vi "HostExample.vi"() -> ()   [LabVIEW 2023]
uses:
  <vilib>/FPGAPlugInAG/Dynamic/niLvFpga_Download_Dynamic.vi
  <vilib>/FPGAPlugInAG/Dynamic/niLvFpga_Run_Dynamic.vi
  <vilib>/LabVIEW Targets/FPGA/RIO/NiFpga_HostInterfaceExtensions/HdlFifo/NiFpga_HdlFifo_AddI32.vi
  API/HdlFifo/private/_NiFpga_HdlFifo_GetStream.vi
  <vilib>/Utility/error.llb/Error Cluster From Error Code.vi
  <vilib>/rvi/interface/nirviMethod/nirviMethod.xnode
  <vilib>/LabVIEW Targets/FPGA/RIO/NiFpga_HostInterfaceExtensions/HdlFifo/NiFpga_HdlFifo_WriteI32.vi
  <vilib>/LabVIEW Targets/FPGA/RIO/NiFpga_HostInterfaceExtensions/HdlFifo/NiFpga_HdlFifo_ReadI32.vi
panel:
  out "empty elements remaining":u64
  out "Elements Remaining":u64
  out "error out 6":errorcluster
  in  "WriteScratch":bool
  in  "ReadScratch":bool
  out "Scratch Read":u32 format="%.0x"
  in  "Scratch Write":u32 format="%.0x"
  in  "Num Elements":i32
  out "Read Data":u32[](array[numeric])
  in  "Read FPGA FIFO":bool
  in  "Write FPGA FIFO":bool
  in  "Write Data":u32[](array[numeric])
  in  "WriteReg":bool
  in  "ReadReg":bool
  out "Read Value":u32
  in  "Write Value":u32 format="%.0x"
  in  "Write Offset":u32
  in  "Read Offset":u32
  in  "Num Elements":i32
  out "Data 4":i32[](array[numeric])
  in  "Write Data":i32[](array[numeric])
  in  "Read Host FIFO":bool
  in  "Write Host FIFO":bool
  out "Numeric":i32
  in  "stop":bool
  # "Write and read any register offset"
  # "Write and read the scratch register"
  # "Scratch Register"
  # "Write and read the Host to FPGA FIFO"
  # "Host to FPGA FIFO"
  # "Write and read the FPGA to Host FIFO"
  # "FPGA to Host FIFO"
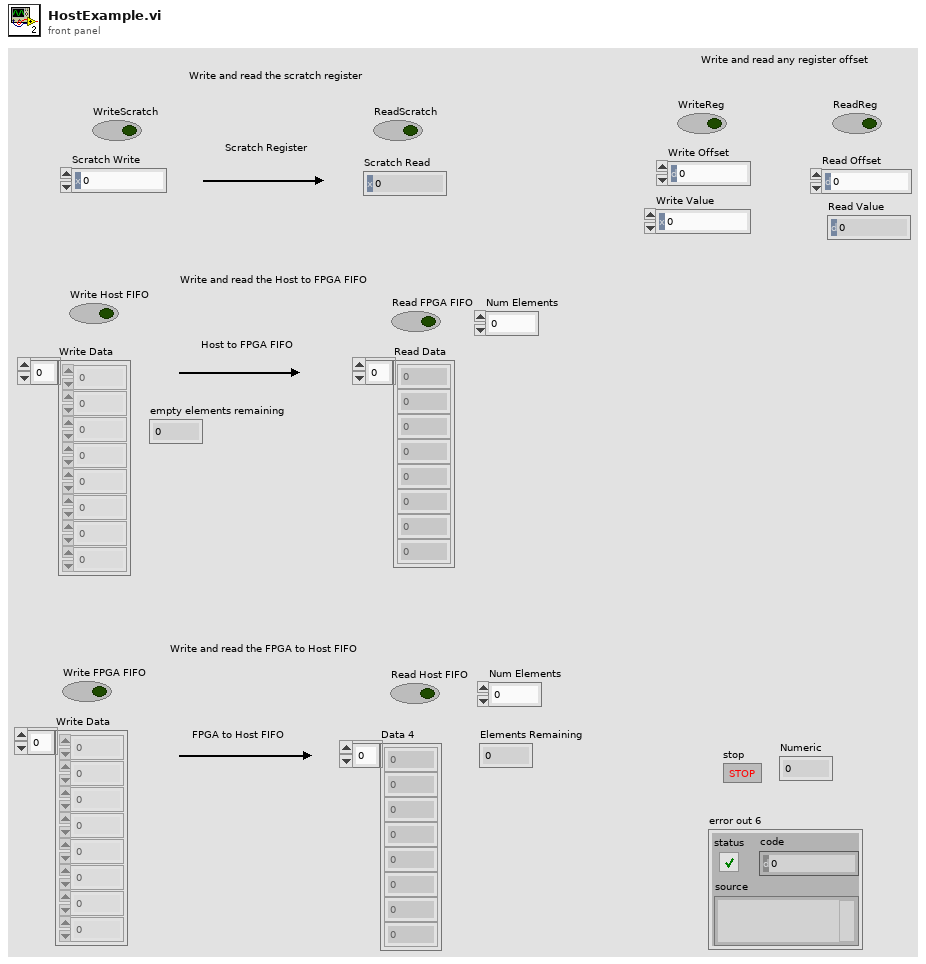
[diagram p1: front panel]
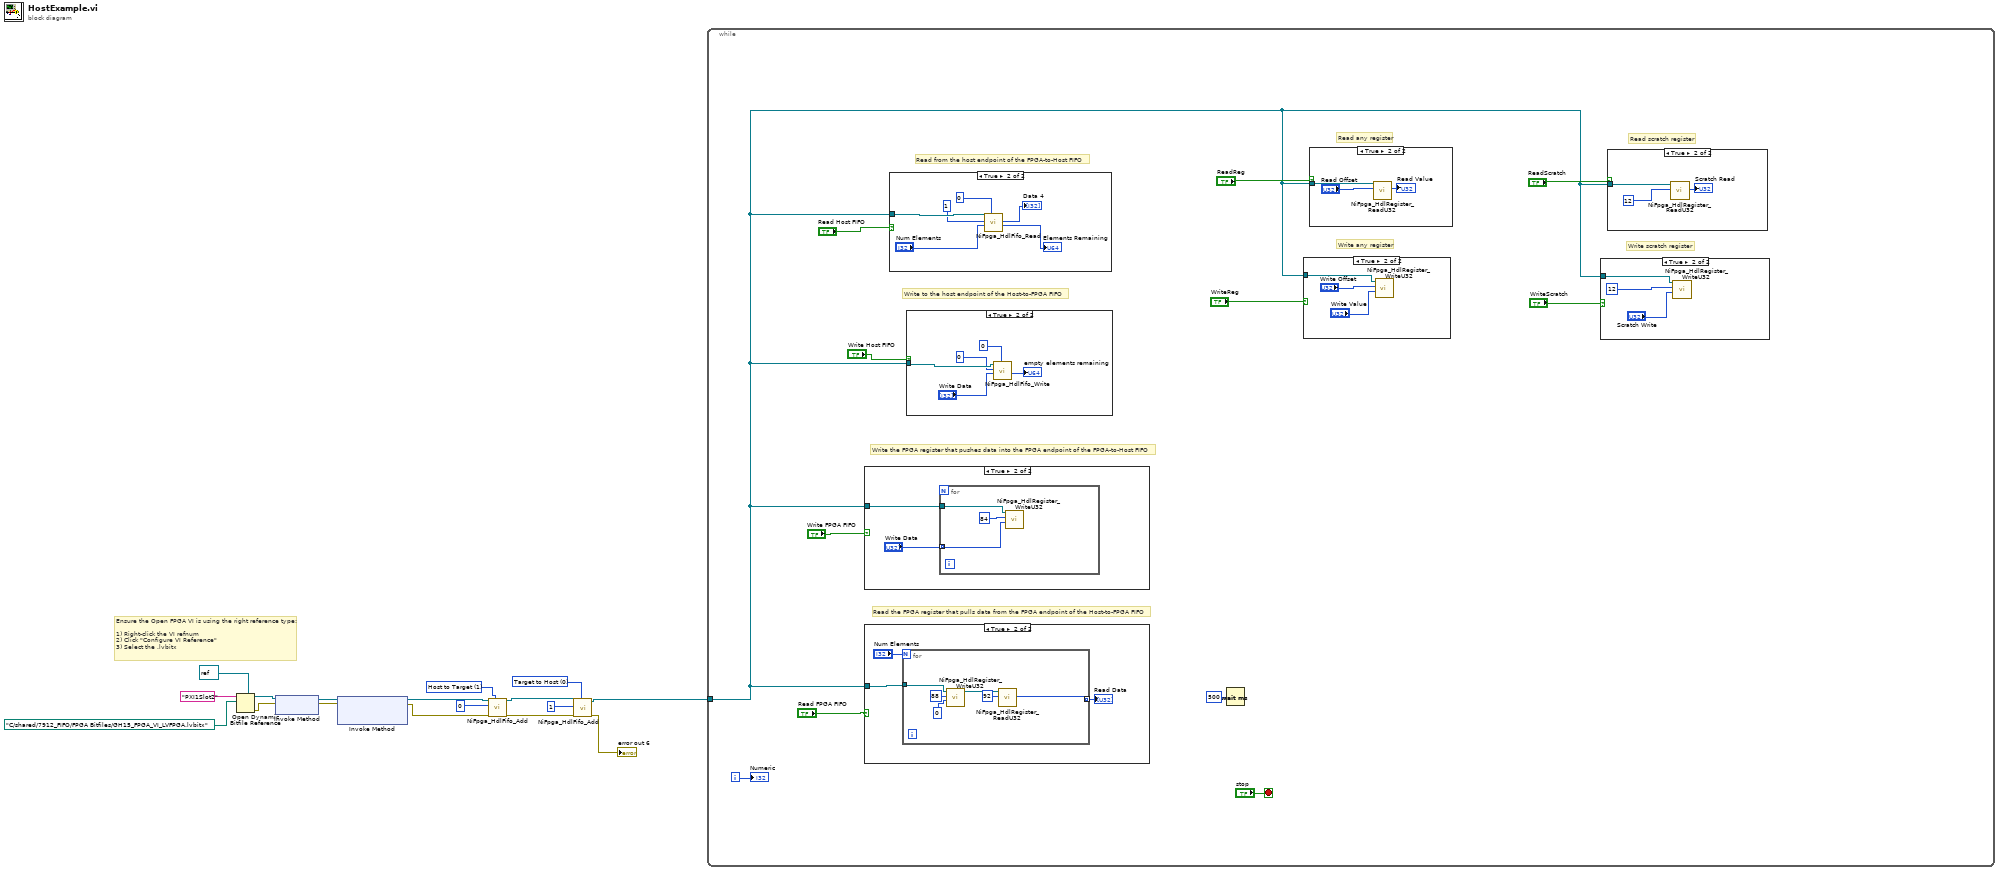
[diagram p0: block diagram]
diagram:
  w2 = u32 0 items=["Target to Host", "Host to Target"] ("direction")
  w9 = u32 1 items=["Target to Host", "Host to Target"]
  # "Ensure the Open FPGA VI is using the right reference type:\n\n1) Right-click the VI refnum \n2) Click \"Configure VI Reference\"\n3) Select the .lvbitx"
  n1 = Open Dynamic Bitfile Reference(0:"PXI1Slot2" ("Device address"), 1:path "C:/shared/7912_FIFO/FPGA Bitfiles/GH15_FPGA_VI_LVFPGA.lvbitx" ("Bitfile path"), 4:refnum<k20> refnum ("Type")) -> (5:w14:refnum<k20>, 8:w13:errorcluster)  [unwired: 2 in]
  n2 = xnode "Invoke Method"("FPGA VI Reference In"=w14, "error in"=w13) -> ("FPGA VI Reference Out"=w16:refnum<k20>, "error out"=w17:errorcluster)
  n3 = xnode "Invoke Method"("FPGA VI Reference In"=w16, "error in"=w17) -> ("FPGA VI Reference Out"=w10:refnum<k20>, "error out"=w4:errorcluster)  [unwired: 1 in]
  n4 = call-poly <vilib>:"NiFpga_HdlFifo_Add.vi"("direction"=w9, "error in (no error)"=w4, "Fifo Number"=u32 0, "FPGA VI Reference In"=w10) -> ("error out"=w1:errorcluster, "FPGA VI Reference Out"=w6:refnum<k20>)  [unwired: 6 in]
  n5 = call-poly <vilib>:"NiFpga_HdlFifo_Add.vi"("direction"=w2, "error in (no error)"=w1, "Fifo Number"=u32 1, "FPGA VI Reference In"=w6) -> ("error out"=→"error out 6":errorcluster, "FPGA VI Reference Out"=w7:refnum<k20>)  [unwired: 6 in]
  n6 = while {
    tunnel: w7 -> [w18]
    i -> [w28]
    stop <- "stop" stop-if-true
    # "Write scratch register"
    # "Read scratch register"
    # "Read any register"
    # "Write any register"
    # "Read from the host endpoint of the FPGA-to-Host FIFO"
    # "Write to the host endpoint of the Host-to-FPGA FIFO"
    # "Read the FPGA register that pulls data from the FPGA endpoint of the Host-to-FPGA FIFO"
    # "Write the FPGA register that pushes data into the FPGA endpoint of the FPGA-to-Host FIFO"
    n7 = case shown="True" "Read FPGA FIFO" {
      tunnel: w18 -> [_ w38]
      frame False {
      }
      frame True {
        n8 = for {
          N: "Num Elements" -> [_]
          tunnel: w38 -> [w44]
          tunnel: [w40] -> w37 mode=indexing
          n9 = call <vilib>:"NiFpga_HdlRegister_WriteU32.vi"("Value"=u32 0, "Offset"=u32 88, "FPGA VI Reference In"=w44) -> ("FPGA VI Reference Out"=w42:refnum<k20>)  [unwired: 6 in, 1 out]
          n10 = call <vilib>:"NiFpga_HdlRegister_ReadU32.vi"("Offset"=u32 92, "FPGA VI Reference In"=w42) -> ("Value"=w40:u32)  [unwired: 7 in, 2 out]
        }
        "Read Data" <- w37
      }
    }
    n11 = case shown="True" "Write FPGA FIFO" {
      tunnel: w18 -> [_ w46]
      frame False {
      }
      frame True {
        n12 = for {
          tunnel: w46 -> [w49]
          tunnel: "Write Data" -> [w47] mode=indexing
          n13 = call <vilib>:"NiFpga_HdlRegister_WriteU32.vi"("Value"=w47, "Offset"=u32 84, "FPGA VI Reference In"=w49) -> ()  [unwired: 6 in, 2 out]
        }
      }
    }
    n14 = case shown="True" "Read Host FIFO" {
      tunnel: w18 -> [_ w65]
      frame False {
      }
      frame True {
        n15 = call-poly <vilib>:"NiFpga_HdlFifo_Read.vi"("timeout"=u32 0, "number of elements"="Num Elements", "fifo number"=u32 1 ("Fifo Number"), "fpga vi reference in"=w65) -> ("elements remaining"=→"Elements Remaining":u64, "data out"=→"Data 4":i32[])  [unwired: 3 in, 2 out]
      }
    }
    n16 = case shown="True" "Write Host FIFO" {
      tunnel: w18 -> [_ w59]
      frame False {
      }
      frame True {
        n17 = call-poly <vilib>:"NiFpga_HdlFifo_Write.vi"("timeout"=u32 0, "data in"="Write Data", "fifo number"=u32 0 ("Fifo Number 2"), "fpga vi reference in"=w59) -> ("empty elements remaining"=→"empty elements remaining":u64)  [unwired: 4 in, 2 out]
      }
    }
    n18 = Wait (ms)(milliseconds to wait=u32 500) -> ()  [unwired: 1 out]
    n19 = case shown="True" "WriteReg" {
      tunnel: w18 -> [_ w52]
      frame False {
      }
      frame True {
        n20 = call <vilib>:"NiFpga_HdlRegister_WriteU32.vi"("Value"="Write Value", "Offset"="Write Offset", "FPGA VI Reference In"=w52) -> ()  [unwired: 6 in, 2 out]
      }
    }
    n21 = case shown="True" "ReadReg" {
      tunnel: w18 -> [_ w55]
      frame False {
      }
      frame True {
        n22 = call <vilib>:"NiFpga_HdlRegister_ReadU32.vi"("Offset"="Read Offset", "FPGA VI Reference In"=w55) -> ("Value"=→"Read Value":u32)  [unwired: 7 in, 2 out]
      }
    }
    n23 = case shown="True" "WriteScratch" {
      tunnel: w18 -> [_ w32]
      frame False {
      }
      frame True {
        n24 = call <vilib>:"NiFpga_HdlRegister_WriteU32.vi"("Value"="Scratch Write", "Offset"=u32 12 ("Write Offset 2"), "FPGA VI Reference In"=w32) -> ()  [unwired: 6 in, 2 out]
      }
    }
    n25 = case shown="True" "ReadScratch" {
      tunnel: w18 -> [_ w35]
      frame False {
      }
      frame True {
        n26 = call <vilib>:"NiFpga_HdlRegister_ReadU32.vi"("Offset"=u32 12 ("Read Offset 2"), "FPGA VI Reference In"=w35) -> ("Value"=→"Scratch Read":u32)  [unwired: 7 in, 2 out]
      }
    }
    "Numeric" <- w28
  }
